vi "Test Panel Template.vi"(7 "Fields In":T1[](array[typedef]), 8 "error in (no error)":errorcluster, 10 "Test Execution Settings":T5={"Quick Mode (T)"=FALSE, "Seq Count"=0, "Step Info"="", "Instruments on Station"=[], "LANGUAGE"="English", "Files Found?"=FALSE, "Step Number"=1} {"Step Number" min=1 step=1}, 11 "Parameters":string) -> (0 "error out":errorcluster, 3 "Test Output":T4, 5 "Fields Out":T1[](array[typedef]))   [LabVIEW 2011]
uses:
  Test Execution Settings.ctl
  typedefs/Instrument Record.ctl
  Test Output.ctl
  typedefs/Field Record.ctl
  typedefs/Field DataTypes.ctl
  typedefs/Field NextItem.ctl
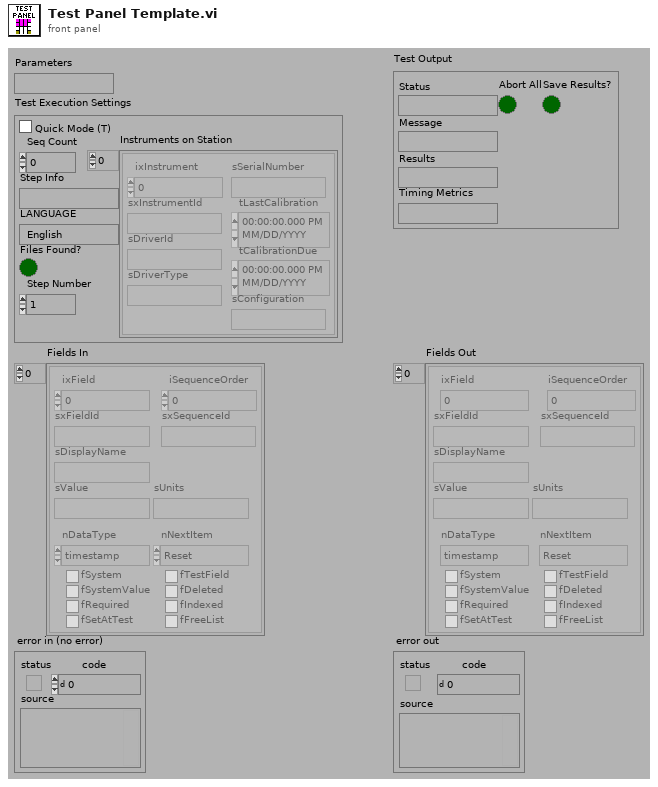
[diagram p1: front panel]
types:
  T1 = typedef "Field Record.ctl" = cluster{"ixField":i32, "iSequenceOrder":i32, "sxFieldId":string, "sxSequenceId":string, "sDisplayName":string, "sValue":string, "sUnits":string, "nDataType":T2, "nNextItem":T3, "fSystem":bool, "fSystemValue":bool, "fRequired":bool, "fSetAtTest":bool, "fTestField":bool, "fDeleted":bool, "fIndexed":bool, "fFreeList":bool}
  T2 = typedef "Field DataTypes.ctl" = enum32{"text", "numeric", "list", "timestamp", "boolean"}
  T3 = typedef "Field NextItem.ctl" = enum32{"Reset", "Retain", "Auto-Increment"}
  T4 = typedef "Test Output.ctl" = cluster{"Status":string, "Message":string, "Results":string, "Abort All":bool, "Save Results?":bool, "Timing Metrics":string}
  T5 = typedef "Test Execution Settings.ctl" = cluster{"Quick Mode (T)":bool, "Seq Count":i32, "Step Info":string, "Instruments on Station":T6[], "LANGUAGE":string, "Files Found?":bool, "Step Number":i32}
  T6 = typedef "Instrument Record.ctl" = cluster{"ixInstrument":i32, "sxInstrumentId":string, "sDriverId":string, "sDriverType":string, "sSerialNumber":string, "tLastCalibration":timestamp, "tCalibrationDue":timestamp, "sConfiguration":string}
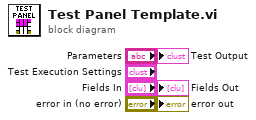
[diagram p0: block diagram]
diagram:
